vi "HMI_OpenFileDialog.vi"(10 "Root Name":string="PWC-OLS", 11 "relative path":path=path "$ReportFiles") -> (0 "selected path":path, 1 "File Name":string, 2 "Root Path":path)   [LabVIEW 2024]
doc: "Use to create relative paths to make the program portable.I\n\niNPUTS\nRelative Path is the name of the folder where to begin the file open dialog.\nRoot Name is the String name of the Root folder of this program.\n\nOUTPUS\nFile Path Path to the Opened File\nRoot Path Path to the root Folder\nFile Name String name less Path and extension."
uses:
  <vilib>/regexp/Match Regular Expression.xnode
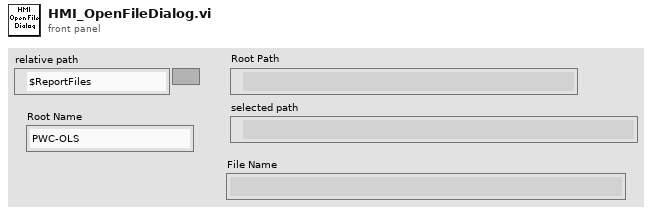
[diagram p1: front panel]
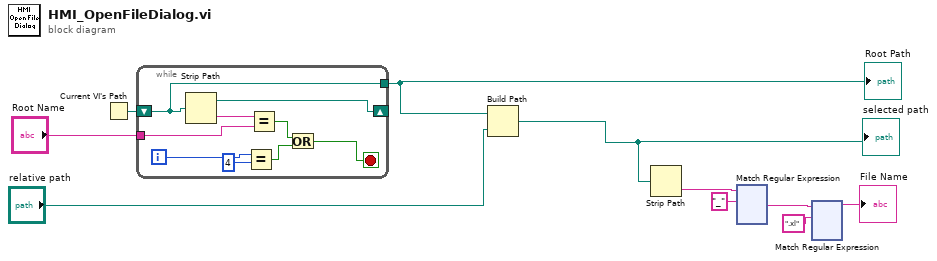
[diagram p0: block diagram]
diagram:
  n1 = Current VI's Path() -> (path=w10:path)
  n2 = while {
    shift-right: [w13] -> _
    shift-left: w10 -> [w12]
    tunnel: [w12] -> w8
    tunnel: "Root Name" -> [w11]
    i -> [w18]
    stop <- w14 stop-if-true
    n3 = Strip Path(path=w12) -> (stripped path=w13:path, name=w19:string)
    n4 = Equal?(x=w18, y=4) -> (x = y?=w15:bool)
    n5 = Equal?(x=w19, y=w11) -> (x = y?=w16:bool)
    n6 = Or(x=w16, y=w15) -> (x .or. y?=w14:bool)
  }
  "Root Path" <- w8
  n7 = Build Path(base path=w8, name or relative path="relative path") -> (appended path=w1:path)
  "selected path" <- w1
  n8 = Strip Path(path=w1) -> (name=w4:string)  [unwired: 1 out]
  n9 = xnode "Match Regular Expression"("input string"=w4, "regular expression"="_") -> ("after match"=w3:string)  [unwired: 4 in, 4 out]
  n10 = xnode "Match Regular Expression"("input string"=w3, "regular expression"=".xl") -> ("before match"=→"File Name":string)  [unwired: 4 in, 4 out]
